vi "Compare If String have same letters.vi"(10 "format string":string, 11 "Letters":string) -> (3 "Same Letters?":bool)   [LabVIEW 2019, in "Day 8.lvlib"]
uses:
  Day 8.lvlib
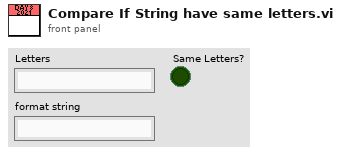
[diagram p1: front panel]
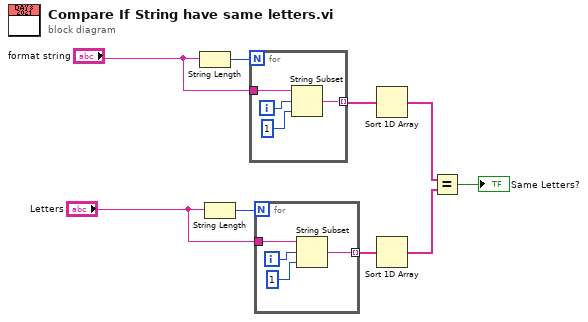
[diagram p0: block diagram]
diagram:
  n1 = String Length(string="format string") -> (length=w8:i32)
  n2 = String Length(string="Letters") -> (length=w7:i32)
  n3 = for {
    N: w8 -> [_]
    tunnel: "format string" -> [w13]
    tunnel: [w10] -> w5 mode=indexing
    i -> [w12]
    n4 = String Subset(string=w13, offset (0)=w12, length (rest)=1 ("length (rest)")) -> (substring=w10:string)
  }
  n5 = for {
    N: w7 -> [_]
    tunnel: "Letters" -> [w17]
    tunnel: [w14] -> w4 mode=indexing
    i -> [w16]
    n6 = String Subset(string=w17, offset (0)=w16, length (rest)=1 ("length (rest)")) -> (substring=w14:string)
  }
  n7 = Sort 1D Array(array=w5) -> (sorted array=w3:string[])
  n8 = Sort 1D Array(array=w4) -> (sorted array=w2:string[])
  n9 = Equal?(x=w3, y=w2) -> (x = y?=→"Same Letters?":bool)
